vi "Bresenhams Line Algorithm.vi"(9 "End":cluster{"X":i32, "Y":i32}, 10 "Start":cluster{"X":i32, "Y":i32}) -> (2 "Line Points":cluster{"X":i32, "Y":i32}[](array[cluster]))   [LabVIEW 2019]
panel:
  # "Bresenham's Line Algorithm calculates the pixels on a line from a given start and end.\nBased upon pseudo-code at http://en.wikipedia.org/wiki/Bresenham%27s_line_algorithm"
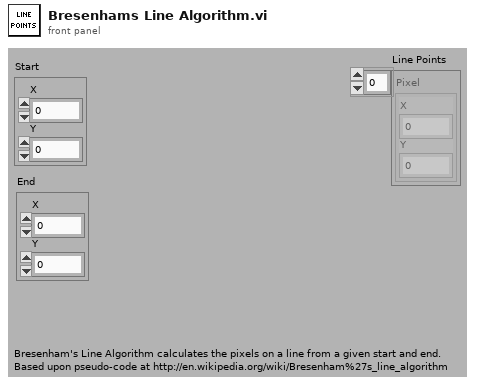
[diagram p1: front panel]
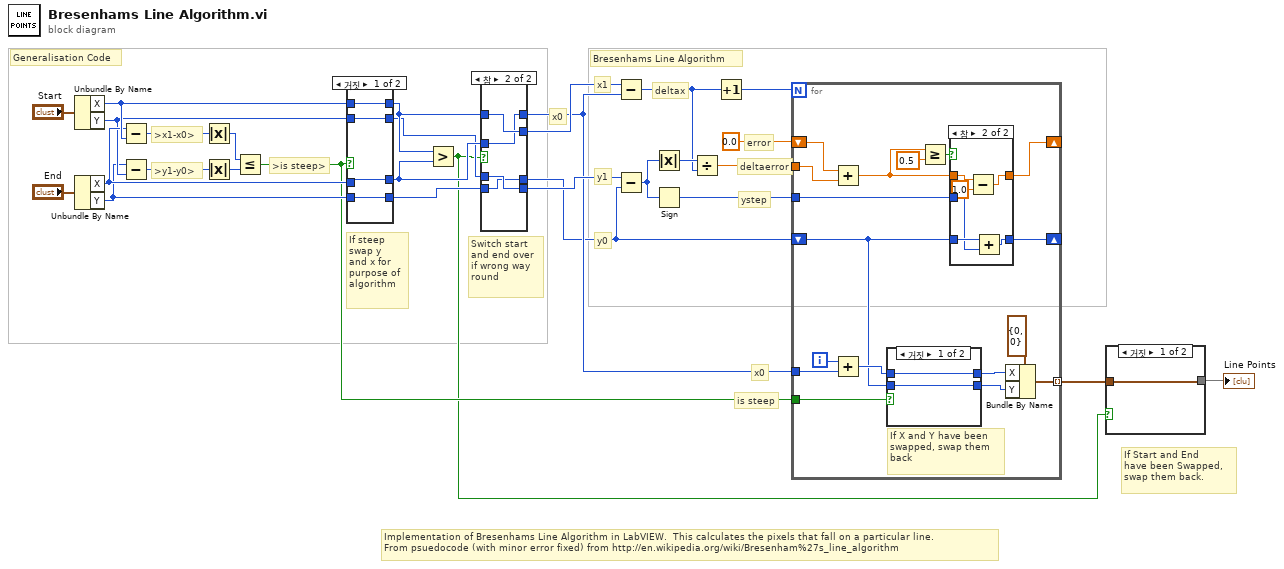
[diagram p0: block diagram]
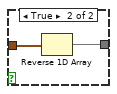
[diagram p2: hidden frame]
diagram:
  # "Bresenhams Line Algorithm"
  # "If Start and End\nhave been Swapped,\nswap them back."
  # "Implementation of Bresenhams Line Algorithm in LabVIEW.  This calculates the pixels that fall on a particular line.\nFrom psuedocode (with minor error fixed) from http://en.wikipedia.org/wiki/Bresenham%27s_line_algorithm"
  # "Switch start\nand end over\nif wrong way\nround"
  # "If steep\nswap y\nand x for\npurpose of\nalgorithm"
  # "is steep"
  # "x0"
  # "Generalisation Code"
  # "y0"
  # "deltaerror"
  # "error"
  # "ystep"
  # "deltax"
  # "y1"
  # "x1"
  # "x0"
  # ">is steep>"
  # ">y1-y0>"
  # ">x1-x0>"
  n1 = Unbundle By Name("Start") -> ("X"=w23:i32, "Y"=w21:i32)
  n2 = Unbundle By Name("End") -> ("X"=w22:i32, "Y"=w20:i32)
  n3 = Subtract(x=w22, y=w23) -> (x-y=w27:i32)
  n4 = Subtract(x=w20, y=w21) -> (x-y=w26:i32)
  n5 = Absolute Value(x=w27) -> (abs(x)=w24:i32)
  n6 = Absolute Value(x=w26) -> (abs(x)=w25:i32)
  n7 = Less Or Equal?(x=w24, y=w25) -> (x <= y?=w6:bool)
  n8 = case shown="거짓" w6 {
    tunnel: w23 -> [w33 w37]
    tunnel: w22 -> [w32 w36]
    tunnel: w21 -> [w31 w35]
    tunnel: w20 -> [w30 w34]
    tunnel: [w31 w37] -> w17
    tunnel: [w30 w36] -> w16
    tunnel: [w33 w35] -> w19
    tunnel: [w32 w34] -> w18
    frame False {
    }
    frame True {
    }
  }
  n9 = Greater?(x=w19, y=w18) -> (0:w3:bool)
  n10 = case shown="참" w3 {
    tunnel: w19 -> [w41 w45]
    tunnel: w18 -> [w40 w44]
    tunnel: w17 -> [w39 w43]
    tunnel: w16 -> [w38 w42]
    tunnel: [w41 w44] -> w11
    tunnel: [w40 w45] -> w15
    tunnel: [w39 w42] -> w8
    tunnel: [w38 w43] -> w14
    frame False {
    }
    frame True {
    }
  }
  n11 = Subtract(x=w15, y=w11) -> (x-y=w5:i32)
  n12 = Subtract(x=w14, y=w8) -> (x-y=w12:i32)
  n13 = Absolute Value(x=w12) -> (abs(x)=w13:i32)
  n14 = Sign(1:w12) -> (0:w7:i32)
  n15 = Divide(x=w13, y=w5) -> (x/y=w9:dbl)
  n16 = Increment(x=w5) -> (x+1=w4:i32)
  n17 = for {
    N: w4 -> [_]
    tunnel: w11 -> [w61]
    shift-right: [w47] -> _
    shift-left: 0.0 -> [w48]
    tunnel: w9 -> [w60]
    tunnel: w7 -> [w50]
    tunnel: w6 -> [w58]
    tunnel: [w54] -> w2 mode=indexing
    shift-right: [w49] -> _
    shift-left: w8 -> [w51]
    i -> [w62]
    # "If X and Y have been\nswapped, swap them\nback"
    n18 = Add(x=w48, y=w60) -> (x+y=w46:dbl)
    n19 = Add(x=w62, y=w61) -> (x+y=w56:i32)
    n20 = case shown="거짓" w58 {
      tunnel: w51 -> [w71 w74]
      tunnel: [w72 w74] -> w57
      tunnel: w56 -> [w72 w73]
      tunnel: [w71 w73] -> w55
      frame False {
      }
      frame True {
      }
    }
    n21 = Greater Or Equal?(x=w46, y=0.5) -> (x >= y?=w53:bool)
    n22 = case shown="참" w53 {
      tunnel: w51 -> [w63 w70]
      tunnel: w50 -> [_ w67]
      tunnel: [w63 w69] -> w49
      tunnel: w46 -> [w64 w68]
      tunnel: [w64 w66] -> w47
      frame False {
      }
      frame True {
        n23 = Subtract(x=w68, y=1.0) -> (x-y=w66:dbl)
        n24 = Add(x=w70, y=w67) -> (x+y=w69:i32)
      }
    }
    n25 = Bundle By Name(cluster=cluster{"X":i32, "Y":i32} {"X"=0, "Y"=0} ("Start"), "X"=w57, "Y"=w55) -> (w54:cluster{"X":i32, "Y":i32})
  }
  n26 = case shown="거짓" w3 {
    tunnel: w2 -> [w75 w77]
    tunnel: [w75 w76] -> w1
    frame False {
    }
    frame True {
      n27 = Reverse 1D Array(array=w77) -> (reversed array=w76:cluster{"X":i32, "Y":i32}[])
    }
  }
  "Line Points" <- w1
